vi "XY Plot.vi"(0 "X":dbl(slide) scale=-1.0..1.0, 1 "X array":dbl[](array[numeric]), 2 "Y array":dbl[](array[numeric]), 3 "Y":dbl(slide) scale=-1.0..1.0, 4 "Angle":dbl format="%#_13g") -> (5 "error":i32, 6 "XY Graph":cluster{"Y":dbl[], "Y":dbl[]}[](graph), 7 "X array":dbl[](array[numeric]), 8 "Y array":dbl[](array[numeric]), 9 "error out":errorcluster)   [LabVIEW 2014]
uses:
  <vilib>/Analysis/coordinate.llb/2D Cartesian Coordinate Rotation (Array).vi
  <vilib>/Analysis/NI_AALPro.lvlib
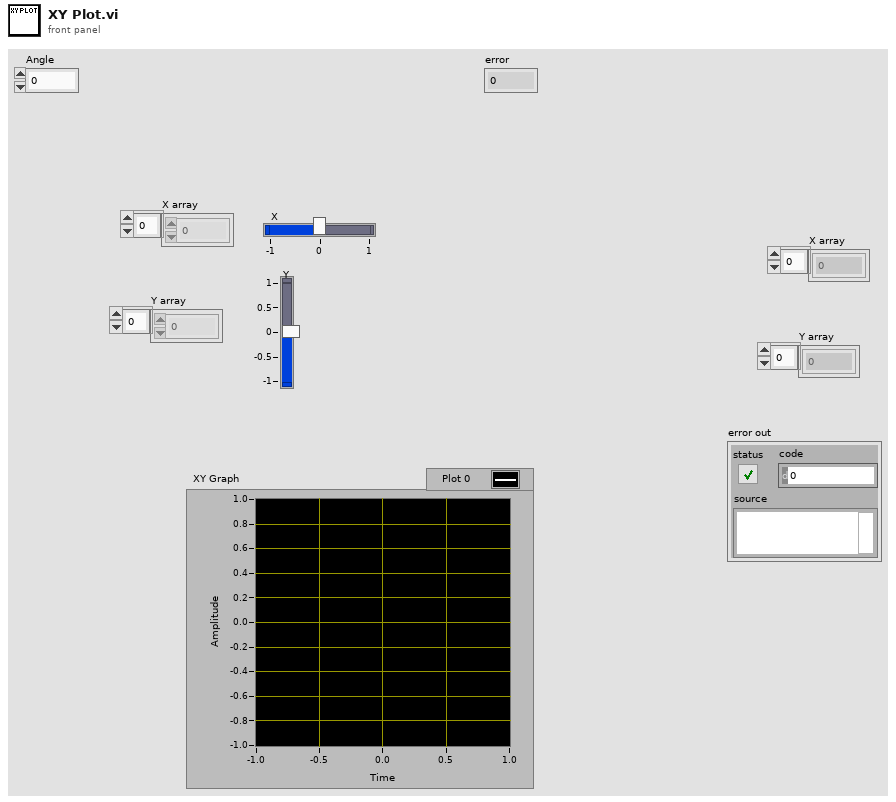
[diagram p1: front panel]
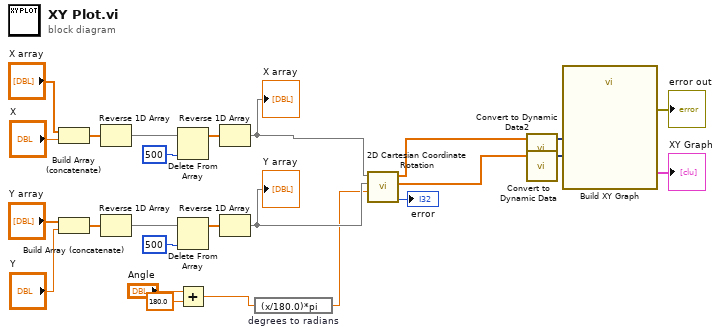
[diagram p0: block diagram]
diagram:
  n1 = Build Array (concatenate)("X array", "X") -> (w19:dbl[])
  n2 = Build Array (concatenate)("Y array", "Y") -> (w17:dbl[])
  n3 = Reverse 1D Array(array=w19) -> (reversed array=w18:dbl[])
  n4 = Reverse 1D Array(array=w17) -> (reversed array=w16:dbl[])
  n5 = Delete From Array(array=w18, index=500) -> (array with subset deleted=w14:dbl[])  [unwired: 1 in, 1 out]
  n6 = Delete From Array(array=w16, index=500) -> (array with subset deleted=w15:dbl[])  [unwired: 1 in, 1 out]
  n7 = Add(x="Angle", y=180.0) -> (x+y=w2:dbl)
  n8 = Reverse 1D Array(array=w14) -> (reversed array=w9:dbl[])
  "X array" <- w9
  n9 = Reverse 1D Array(array=w15) -> (reversed array=w11:dbl[])
  "Y array" <- w11
  n10 = expression code="(x/180.0)*pi" "degrees to radians"(w2) -> (w1:dbl)
  n11 = call-poly <vilib>:"2D Cartesian Coordinate Rotation.vi"("theta"=w1, "Y"=w11, "X"=w9) -> ("error"=→"error":i32, "Y Out"=w6:dbl[], "X Out"=w7:dbl[])  [unwired: 6 in]
  n12 = call "Convert to Dynamic Data2"("Array"=w7) -> ("Dynamic Data Type"=w8:dynamicdata)  [unwired: 3 in]
  n13 = call "Convert to Dynamic Data"("Array"=w6) -> ("Dynamic Data Type"=w10:dynamicdata)  [unwired: 3 in]
  n14 = call "Build XY Graph"("Y Input"=w10, "X Input"=w8) -> ("error out"=→"error out":errorcluster, "XY Graph"=→"XY Graph":cluster{"X":dbl[], "Y":dbl[]}[])  [unwired: 8 in]
